vi "Force Square Scale.vi"(8 "error in (no error)":errorcluster, 11 "Plot Area Ref":refnum<vi>) -> (0 "error out":errorcluster)   [LabVIEW 2017, in "2D Compass.lvclass"]
uses:
  <vilib>/Math Plots/2D Math Plots/2D Compass/2D Compass/2D Compass.lvclass
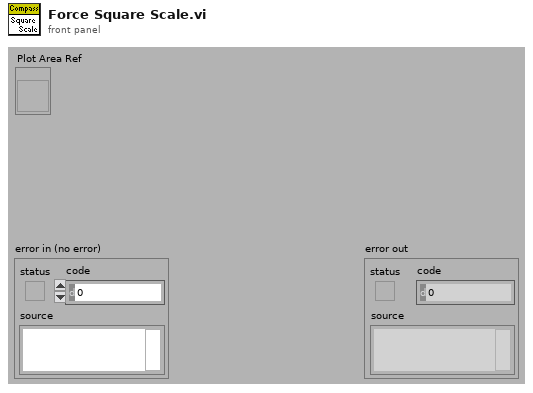
[diagram p1: front panel]
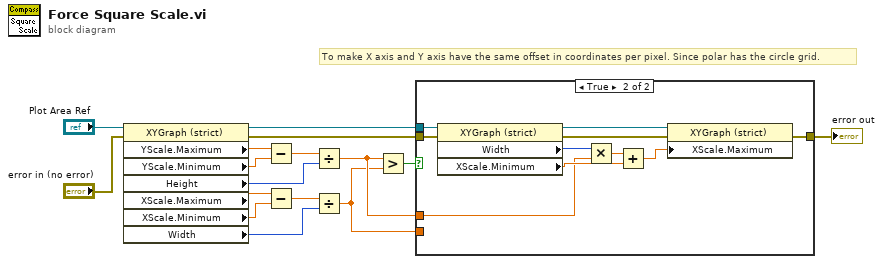
[diagram p0: block diagram]
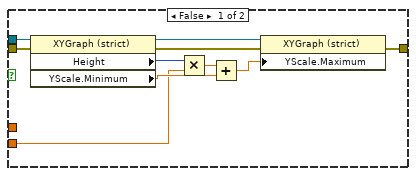
[diagram p2: hidden frame]
diagram:
  # "To make X axis and Y axis have the same offset in coordinates per pixel. Since polar has the circle grid."
  n1 = property on="Property Node" class="XYGraph (strict)"(reference="Plot Area Ref", error in="error in (no error)") -> (reference out=w15:refnum<vi>, error out=w14:errorcluster, "YScale.Maximum"=w12:dbl, "YScale.Minimum"=w13:dbl, "Height"=w10:u32, "XScale.Maximum"=w9:dbl, "XScale.Minimum"=w8:dbl, "Width"=w6:u32)
  n2 = Subtract(x=w12, y=w13) -> (x-y=w11:dbl)
  n3 = Subtract(x=w9, y=w8) -> (x-y=w7:dbl)
  n4 = Divide(x=w11, y=w10) -> (x/y=w4:dbl)
  n5 = Divide(x=w7, y=w6) -> (x/y=w3:dbl)
  n6 = Greater?(x=w4, y=w3) -> (0:w5:bool)
  n7 = case shown="True" w5 {
    tunnel: [w17 w32] -> w16
    tunnel: w15 -> [w20 w31]
    tunnel: w14 -> [w19 w30]
    tunnel: w4 -> [_ w29]
    tunnel: w3 -> [w18 _]
    frame False {
      n8 = property on="Property Node" class="XYGraph (strict)"(reference=w20, error in=w19) -> (reference out=w26:refnum<vi>, error out=w21:errorcluster, "Height"=w22:u32, "YScale.Minimum"=w24:dbl)
      n9 = Multiply(x=w22, y=w18) -> (x*y=w25:dbl)
      n10 = Add(x=w25, y=w24) -> (x+y=w23:dbl)
      n11 = property on="Property Node" class="XYGraph (strict)"(reference=w26, error in=w21, "YScale.Maximum"=w23) -> (error out=w17:errorcluster)  [unwired: 1 out]
    }
    frame True {
      n12 = property on="Property Node" class="XYGraph (strict)"(reference=w31, error in=w30) -> (reference out=w36:refnum<vi>, error out=w27:errorcluster, "Width"=w28:u32, "XScale.Minimum"=w34:dbl)
      n13 = Multiply(x=w28, y=w29) -> (x*y=w35:dbl)
      n14 = Add(x=w35, y=w34) -> (x+y=w33:dbl)
      n15 = property on="Property Node" class="XYGraph (strict)"(reference=w36, error in=w27, "XScale.Maximum"=w33) -> (error out=w32:errorcluster)  [unwired: 1 out]
    }
  }
  "error out" <- w16
